vi "TAI_Servo.vi"(2 "Normal Output":dbl, 3 "Actuator Name":string) -> (0 "Interlock Output":dbl, 1 "Testing This Actuator":bool)   [LabVIEW 2019]
doc: "This VI is configured for polymorphic use and functions as an interlock, allowing the selected servo to be tested manually via the FRC 4265 Dashboard. During testing, all interlocked actuators which are not selected for testing are disabled."
uses:
  dsdata.vi
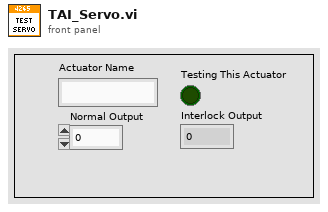
[diagram p1: front panel]
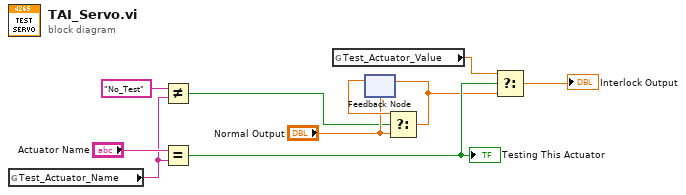
[diagram p0: block diagram]
diagram:
  n1 = global read "dsdata.vi" "Test_Actuator_Name"() -> (w8:string)
  n2 = Not Equal?(x="No_Test", y=w8) -> (x != y?=w2:bool)
  n3 = Equal?(x="Actuator Name", y=w8) -> (x = y?=w6:bool)
  "Testing This Actuator" <- w6
  n4 = global read "dsdata.vi" "Test_Actuator_Value"() -> (w7:dbl)
  n5 = feedback #1("Normal Output") -> (w4:dbl)
  n6 = Select(t=w4, s=w2, f="Normal Output") -> (s? t:f=w1:dbl)
  n7 = feedback-in #1(w1) -> ()
  n8 = Select(t=w7, s=w6, f=w1) -> (s? t:f=→"Interlock Output":dbl)
